vi "Test Invalid Registration - Bad Flow Name.vi"() -> ()   [LabVIEW 2024]
uses:
  Sift API/Sift Client.lvclass
  Generate Sift Protos/SiftProxy_client/RPC Messages/sift_proxy_v1_ChannelDataType.ctl
  Generate Sift Protos/SiftProxy_client/SiftProxy_client.lvlib
  Generate Sift Protos/SiftProxy_client/RPC Messages/sift_proxy_v1_ChannelBitFieldElement_Flat.ctl
  Generate Sift Protos/SiftProxy_client/RPC Messages/sift_proxy_v1_ChannelEnumType_Flat.ctl
  Generate Sift Protos/SiftProxy_client/RPC Messages/sift_proxy_v1_ChannelConfig_Flat.ctl
panel:
  out "Success":bool
  in  "sift_proxy_v1_ChannelConfig_Flat":T1
  out "Error":errorcluster
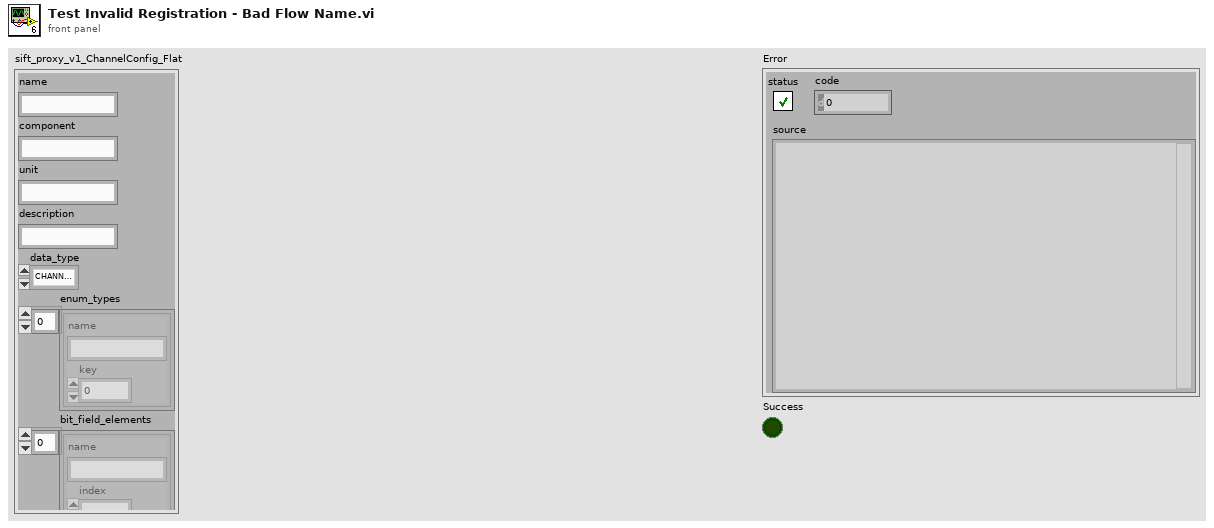
[diagram p1: front panel]
types:
  T1 = typedef "SiftProxy_client.lvlib/sift_proxy_v1_ChannelConfig_Flat.ctl" = cluster{"name":string, "component":string, "unit":string, "description":string, "data_type":T2, "enum_types":T3[], "bit_field_elements":T4[]}
  T2 = typedef "SiftProxy_client.lvlib/sift_proxy_v1_ChannelDataType.ctl" = enum32{"CHANNEL_DATA_TYPE_UNSPECIFIED", "CHANNEL_DATA_TYPE_DOUBLE", "CHANNEL_DATA_TYPE_STRING", "CHANNEL_DATA_TYPE_ENUM", "CHANNEL_DATA_TYPE_BIT_FIELD", "CHANNEL_DATA_TYPE_BOOL", "CHANNEL_DATA_TYPE_FLOAT", "CHANNEL_DATA_TYPE_INT_32", "CHANNEL_DATA_TYPE_UINT_32", "CHANNEL_DATA_TYPE_INT_64", "CHANNEL_DATA_TYPE_UINT_64"}
  T3 = typedef "SiftProxy_client.lvlib/sift_proxy_v1_ChannelEnumType_Flat.ctl" = cluster{"name":string, "key":u32}
  T4 = typedef "SiftProxy_client.lvlib/sift_proxy_v1_ChannelBitFieldElement_Flat.ctl" = cluster{"name":string, "index":i32, "bit_count":u32}
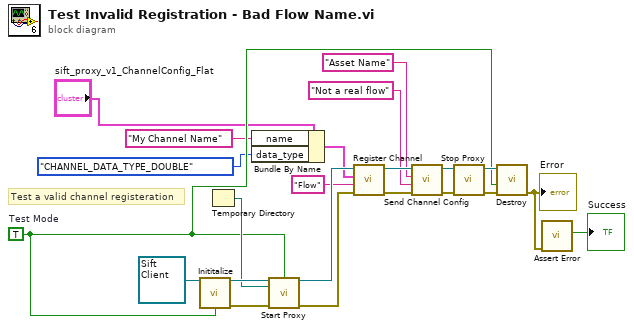
[diagram p0: block diagram]
diagram:
  w16 = TRUE  # Test Mode
  # "Test a valid channel registeration"
  n1 = call-dynamic "Inititalize.vi"("Sift Client in"=refnum<class "Sift Client.lvclass"> refnum ("Sift Client.lvlib:Sift Client.lvclass"), "Test Mode"=w16) -> ("Sift Client out"=w21:refnum<class "Sift Client.lvclass">, "error out"=w20:errorcluster)  [unwired: 12 in]
  n2 = Temporary Directory() -> (w17:path)
  n3 = Bundle By Name(cluster="sift_proxy_v1_ChannelConfig_Flat", "name"="My Channel Name", "data_type"=sift_proxy_v1_ChannelDataType."CHANNEL_DATA_TYPE_DOUBLE" ("sift_proxy_v1_ChannelDataType")) -> (w11:T1)
  n4 = call-dynamic "Start Proxy.vi"("Sift Client in"=w21, "Test Mode"=w16, "Storage Path"=w17, "error in (no error)"=w20) -> ("Sift Client out"=w15:refnum<class "Sift Client.lvclass">, "error out"=w10:errorcluster)  [unwired: 10 in]
  n5 = call-dynamic "Register Channel.vi"("error in (no error)"=w10, "Flow Name"="Flow", "Channel Config"=w11, "Sift Client in"=w15) -> ("error out"=w6:errorcluster, "Sift Client out"=w8:refnum<class "Sift Client.lvclass">)  [unwired: 6 in]
  n6 = call-dynamic "Send Channel Config.vi"("error in (no error)"=w6, "Flow Name"="Not a real flow", "Asset Name"="Asset Name", "Sift Client in"=w8) -> ("error out"=w4:errorcluster, "Sift Client out"=w5:refnum<class "Sift Client.lvclass">)  [unwired: 6 in]
  n7 = call-dynamic "Stop Proxy.vi"("error in (no error)"=w4, "Sift Client in"=w5) -> ("error out"=w19:errorcluster, "Sift Client out"=w18:refnum<class "Sift Client.lvclass">)  [unwired: 7 in, 1 out]
  n8 = call-dynamic "Destroy.vi"("error in (no error)"=w19, "Test Mode"=w16, "Sift Client in"=w18) -> ("error out"=w2:errorcluster)  [unwired: 7 in, 1 out]
  "Error" <- w2
  n9 = call "Assert Error.vi"("Error"=w2) -> ("Success"=→"Success":bool)  [unwired: 10 in]
